vi "Resize Window.vi"(8 "error in":errorcluster caption="error in (no error)" {"code" format="%d\n%x"}, 9 "new Size":cluster{"Width":i32, "Height":i32}, 10 "window name (\"\")":string, 11 "window refnum":T1 caption="window refnum (NaWR)") -> (0 "error out":errorcluster {"code" format="%d\n%x"}, 1 "prev size":cluster{"Width":i16, "Height":i16}, 3 "window refnum out":T1)   [LabVIEW 2020, in "MacroAssert.lvlib" / "Win Util New.lvlib"]
doc: "This function will resize (without moving) the window named in the window name input or identified by the window refnum. Window size is determined in pixels. If the window cannot be found, an error will be returned."
uses:
  Win Util New.lvlib
  Window Refnum.ctl
  user32.dll
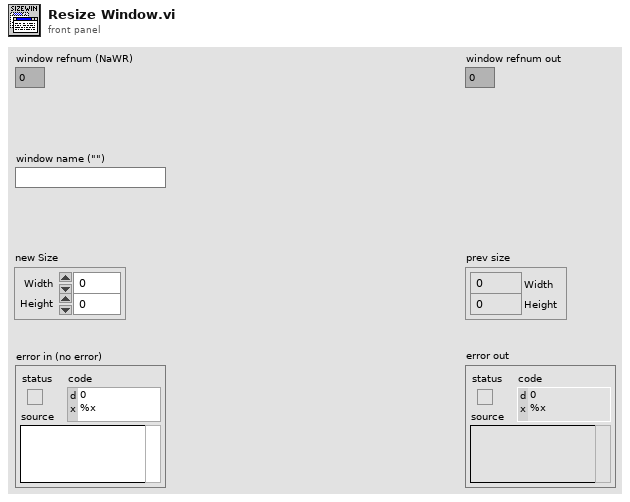
[diagram p1: front panel]
types:
  T1 = typedef "MacroAssert.lvlib/Win Util New.lvlib/Window Refnum.ctl" = u64
  T2 = cluster{"left":i16, "top":i16, "right":i16, "bottom":i16}
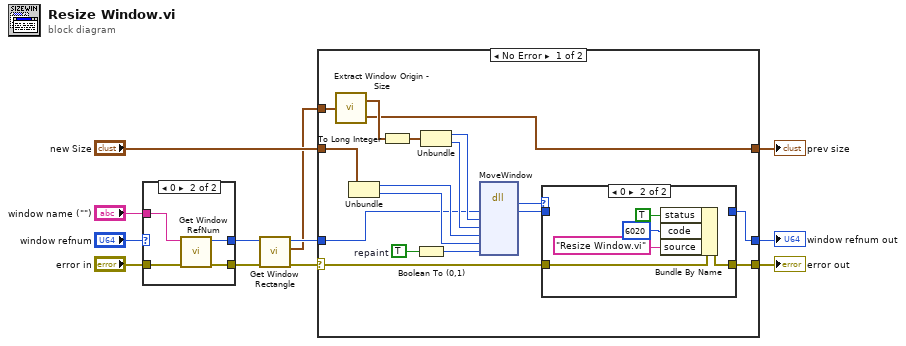
[diagram p0: block diagram]
diagram:
  n1 = case shown="0" "window refnum" {
    selector: "window refnum" -> [w13 _]
    tunnel: "error in" -> [w14 w18]
    tunnel: [w13 w17] -> w8
    tunnel: [w14 w16] -> w9
    tunnel: "window name (\"\")" -> [_ w15]
    frame Default {
    }
    frame 0 {
      n2 = call "Get Window RefNum.vi"("error in"=w18, "window name (\"\")"=w15) -> ("error out"=w16:errorcluster, "window refnum (NaWR)"=w17:T1)  [unwired: 6 in]
    }
  }
  n3 = call "Get Window Rectangle.vi"("error in"=w9, "window refnum (NaWR)"=w8) -> ("error out"=w3:errorcluster, "window rect"=w1:T2, "window refnum out"=w11:T1)  [unwired: 7 in]
  n4 = case shown="No Error" w3 {
    selector: w3 -> [w23 w44]
    tunnel: w1 -> [w35 _]
    tunnel: [w24 w44] -> w12
    tunnel: w11 -> [w26 w45]
    tunnel: [w22 w45] -> w10
    tunnel: "new Size" -> [w27 w43]
    tunnel: [w25 w43] -> w2
    frame No Error {
      w34 = TRUE  # repaint
      n5 = call "Extract Window Origin - Size.vi"("window rect"=w35) -> ("window origin"=w32:cluster{"left":i16, "top":i16}, "window size"=w25:cluster{"Width":i16, "Height":i16})
      n6 = Unbundle(w27) -> ("Width"=w29:i32, "Height"=w28:i32)
      n7 = To Long Integer(number=w32) -> (32bit integer=w19:cluster{"left":i32, "top":i32})
      n8 = Boolean To (0,1)(Boolean=w34) -> (0, 1=w33:i16)
      n9 = Unbundle(w19) -> ("left"=w31:i32, "top"=w30:i32)
      n10 = dll-call lib="USER32.DLL" fn="MoveWindow"("hWnd"=w26, "left"=w31, "top"=w30, "right"=w29, "bottom"=w28, "repaint"=w33) -> ("error"=w21:i32, "hWnd"=w20:u64)  [unwired: 3 in, 7 out]
      n11 = case shown="0" w21 {
        tunnel: [w37 w42] -> w24
        tunnel: w23 -> [w37 w41]
        tunnel: [w36 _] -> w22
        tunnel: w20 -> [w36 _]
        frame Default {
        }
        frame 0 {
          n12 = Bundle By Name(cluster=w41, "status"=TRUE, "code"=6020, "source"="Resize Window.vi") -> (w42:errorcluster)
        }
      }
    }
    frame Error {
    }
  }
  "error out" <- w12
  "window refnum out" <- w10
  "prev size" <- w2
